vi "pH_Sensor_Calibration.vi"(11 "read_in":dbl format="%0.2f") -> (2 "pH value":dbl, 3 "pH":dbl(knob) scale=0.0..14.0)   [LabVIEW 2022 SP3]
uses:
  <vilib>/ptbypt/NI_PtbyPt.lvlib
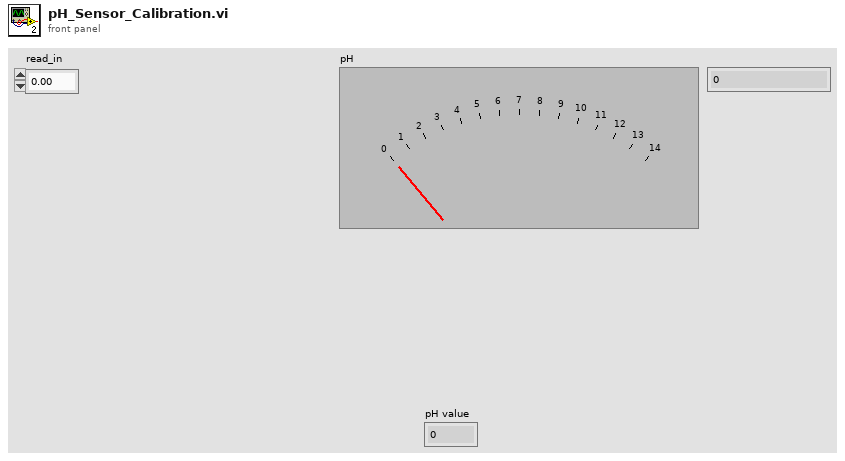
[diagram p1: front panel]
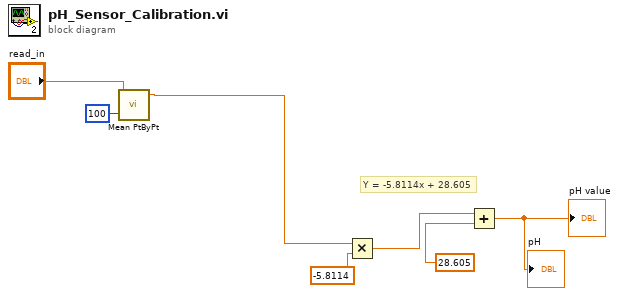
[diagram p0: block diagram]
diagram:
  # "Y = -5.8114x + 28.605"
  n1 = call <vilib>:"Mean PtByPt.vi"("x"="read_in", "sample length"=100) -> ("mean"=w4:dbl)  [unwired: 2 in, 1 out]
  n2 = Multiply(x=w4, y=-5.8114) -> (x*y=w3:dbl)
  n3 = Add(x=w3, y=28.605) -> (x+y=→"pH" →"pH value":dbl)
